vi "DHE_SetPrePostNumFrames.vi"(2 "DHE_PreExpose":i32, 3 "DHE_PostExpose":i32) -> ()   [LabVIEW 2016]
uses:
  private/vis/DHE_GBLDriverVariables.vi
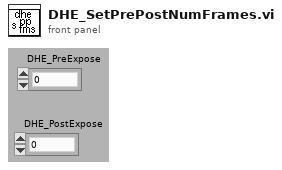
[diagram p1: front panel]
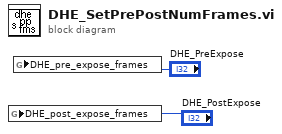
[diagram p0: block diagram]
diagram:
  n1 = global write "DHE_GBLDriverVariables.vi" "DHE_post_expose_frames"("DHE_PostExpose") -> ()
  n2 = global write "DHE_GBLDriverVariables.vi" "DHE_pre_expose_frames"("DHE_PreExpose") -> ()
